vi "ini udp stream.vi"(9 "UDP Port":u16, 10 "UDP IP Port":string) -> (0 "error out udp":errorcluster, 3 "connection ID":refnum<k16>)   [LabVIEW 2021]
uses:
  <vilib>/Utility/tcp.llb/UDP Multicast Read-Write Open.vi
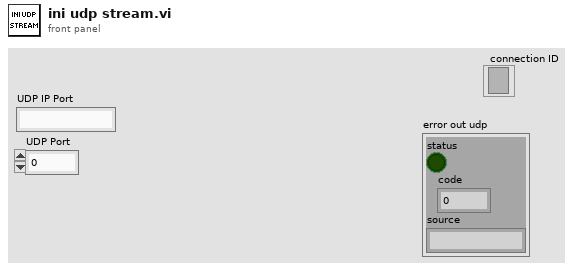
[diagram p1: front panel]
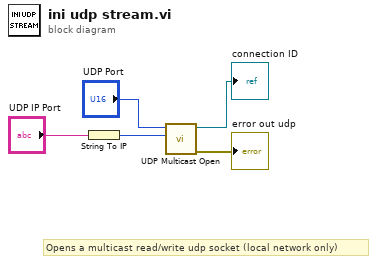
[diagram p0: block diagram]
diagram:
  # "Opens a multicast read/write udp socket (local network only)"
  n1 = String To IP(1:"UDP IP Port") -> (0:w2:u32)
  n2 = call-poly <vilib>:"UDP Multicast Open.vi"("multicast addr"=w2, "port"="UDP Port") -> ("error out"=→"error out udp":errorcluster, "connection ID"=→"connection ID":refnum<k16>)  [unwired: 7 in, 1 out]
